vi "(Depricated) Dialog Sample.vi"(7 "Sample Line Control Ref":refnum<vi>, 8 "Error In":errorcluster, 11 "Caller-To-Actor Enqueuer":refnum<class "Message Enqueuer.lvclass">) -> (0 "Error Out":errorcluster, 1 "Sample Removed":bool, 3 "Cancelled?":bool)   [LabVIEW 2015]
doc: "Use this template to create a dialog box with event handling."
uses:
  <vilib>/ActorFramework/Message Enqueuer/Message Enqueuer.lvclass
  Controls/Ti Colors.ctl
panel:
  out "Color Box":u32(colorbox)
  in  "Remove Button":bool
  in  "Comment":string
  in  "Ti Cathode":i8 min=-1 max=39 step=1
  in  "Sample Name":string
  in  "Cancel":bool
  in  "OK":bool
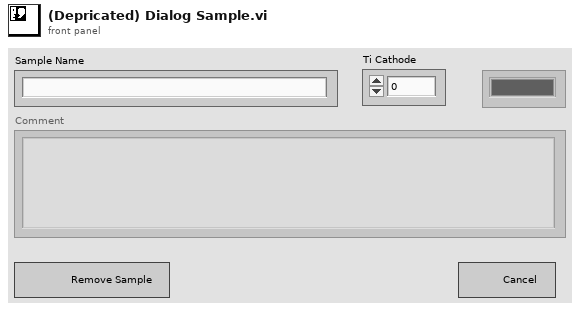
[diagram p1: front panel]
types:
  T1 = typedef "Ti Colors.ctl" = u32[]
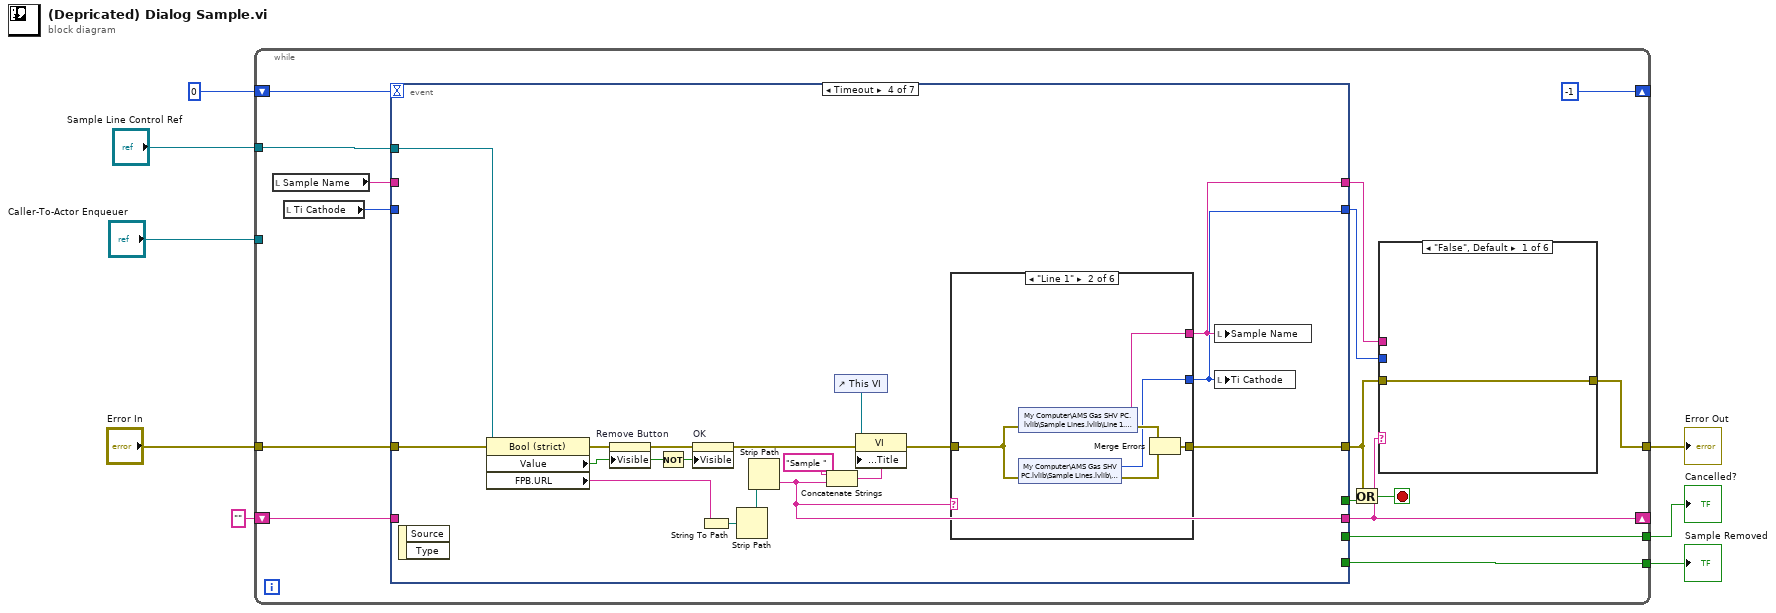
[diagram p0: block diagram]
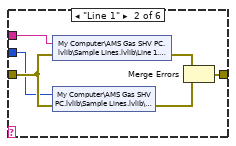
[diagram p2: hidden frame]
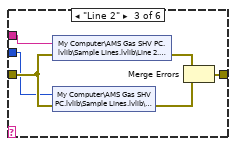
[diagram p3: hidden frame]
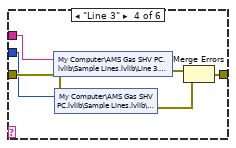
[diagram p4: hidden frame]
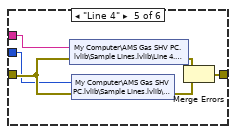
[diagram p5: hidden frame]
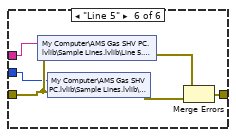
[diagram p6: hidden frame]
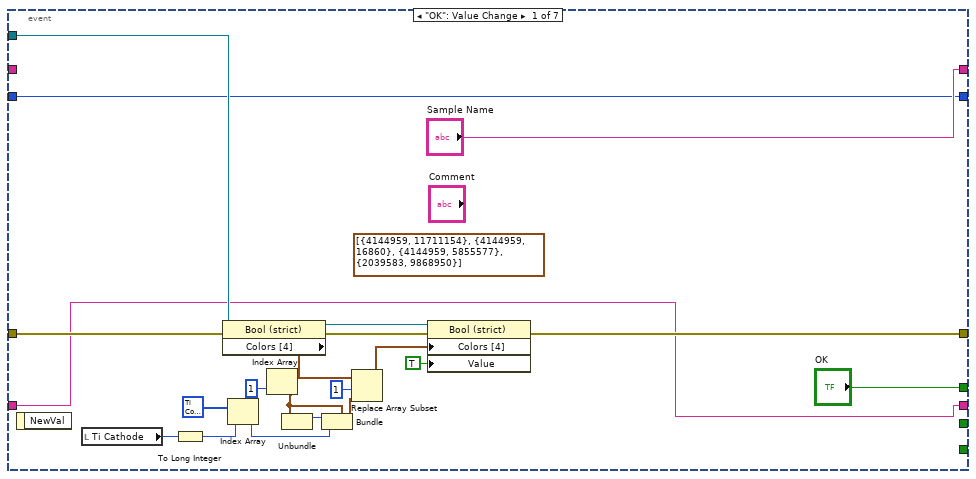
[diagram p7: hidden frame]
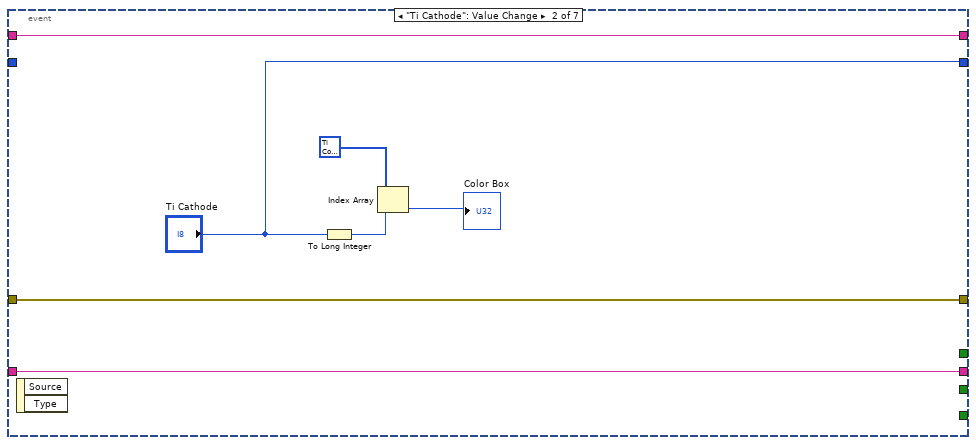
[diagram p8: hidden frame]
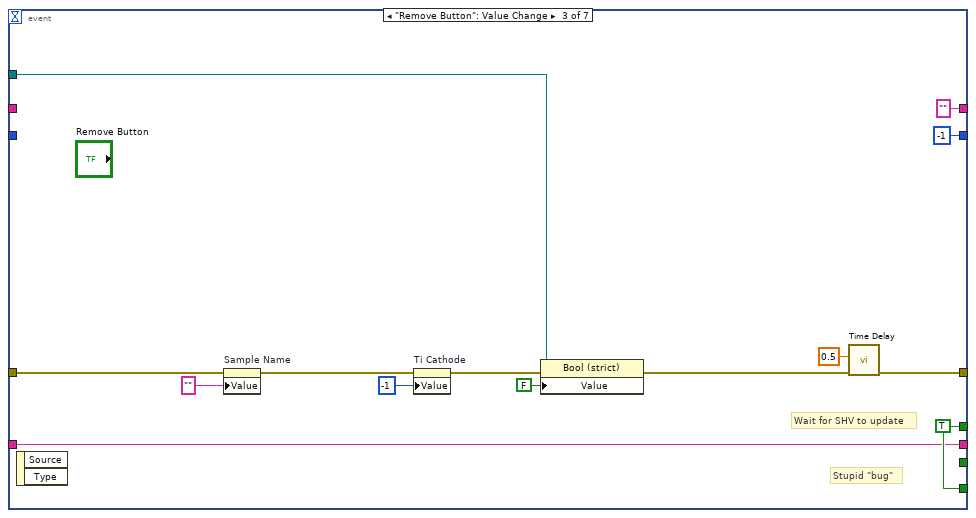
[diagram p9: hidden frame]
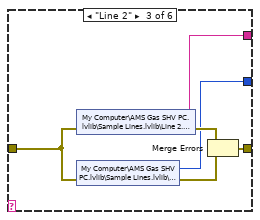
[diagram p11: hidden frame]
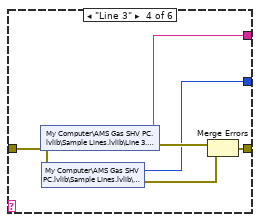
[diagram p12: hidden frame]
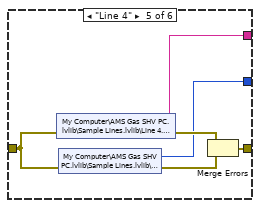
[diagram p13: hidden frame]
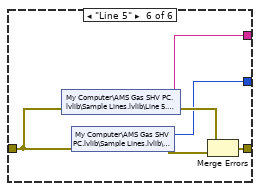
[diagram p14: hidden frame]
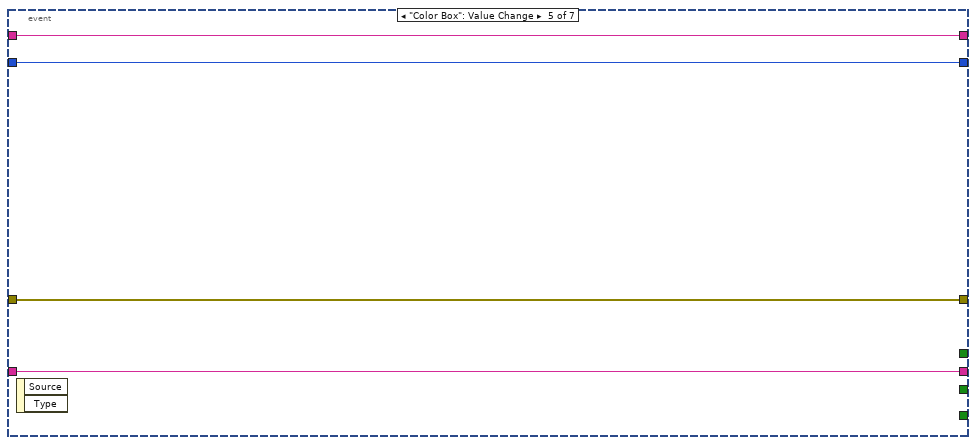
[diagram p15: hidden frame]
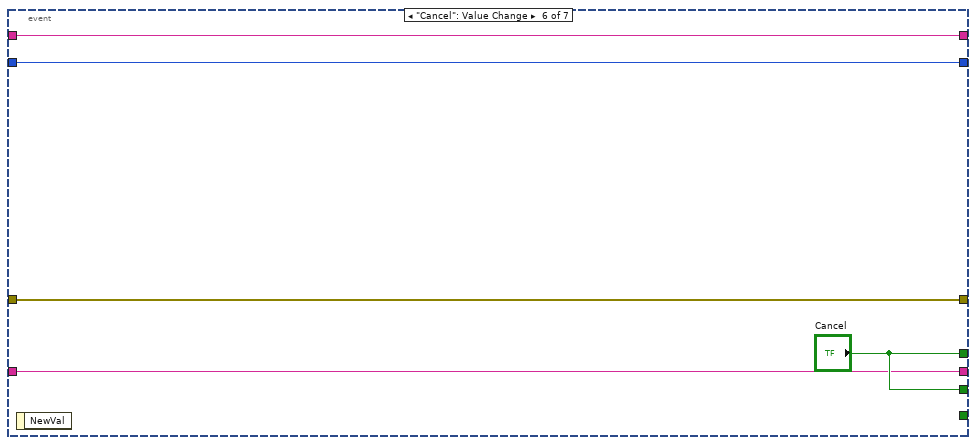
[diagram p16: hidden frame]
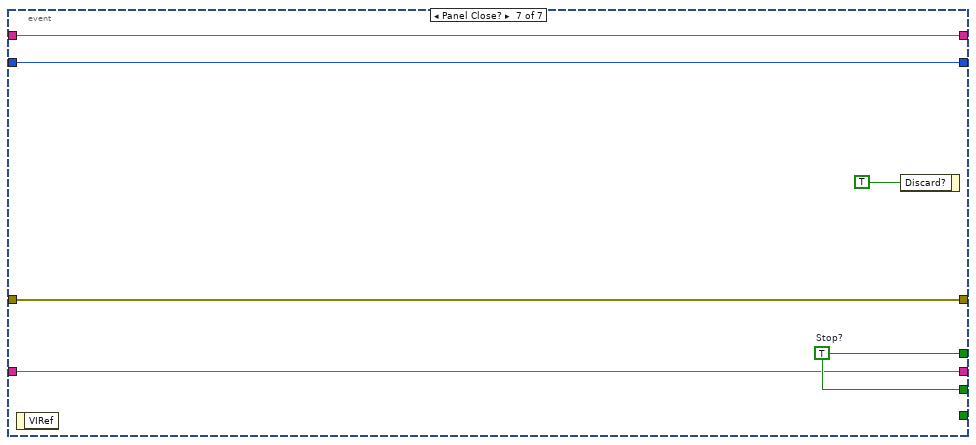
[diagram p17: hidden frame]
diagram:
  n1 = while {
    tunnel: "Error In" -> [w24]
    tunnel: "Caller-To-Actor Enqueuer" -> [_]
    tunnel: [w15] -> w7
    tunnel: "Sample Line Control Ref" -> [w23]
    shift-right: [-1] -> _
    shift-left: 0 -> [w20]
    tunnel: [w19] -> w4
    tunnel: [w17] -> w2
    shift-right: [w14] -> _
    shift-left: "" ("name") -> [w13]
    stop <- w21 stop-if-true
    n2 = local read "Sample Name"() -> (w12:string)
    n3 = local read "Ti Cathode"() -> (w11:i8)
    n4 = event shown="[3] Timeout" {
      selector: _ -> [_ _ _ _ _ _ _]
      dyn-events: _ -> [_ _ _ _ _ _ _]
      timeout: w20 -> [_ _ _ _ _ _ _]
      tunnel: ["OK" _ w89 _ _ "Cancel" w158] -> w22
      tunnel: w24 -> [w73 w80 w92 w112 w149 w154 w159]
      tunnel: [w75 w80 w94 w101 w149 w154 w159] -> w16
      tunnel: w23 -> [w71 _ w97 w113 _ _ _]
      tunnel: [_ _ _ _ _ "Cancel" w158] -> w19
      tunnel: [_ _ w89 _ _ _ _] -> w17
      tunnel: [w61 w79 w86 w100 w148 w152 w157] -> w14
      tunnel: w13 -> [w61 w79 w86 _ w148 w152 w157]
      tunnel: w12 -> [_ w78 _ _ w147 w151 w156]
      tunnel: w11 -> [w59 _ _ _ w146 w150 w155]
      tunnel: ["Sample Name" w78 "" ("Sample Name") w99 w147 w151 w156] -> w10
      tunnel: [w59 "Ti Cathode" i8 -1 ("Ti Cathode") w98 w146 w150 w155] -> w9
      event "OK": Value Change {
        (unwired) cluster{u32, u32}[] [{4144959, 11711154}, {4144959, 16860}, {4144959, 5855577}, {2039583, 9868950}] ("Colors [4]")
        n5 = event-data() -> ()  [unwired: 1 in, 1 out]
        n6 = local read "Ti Cathode"() -> (w65:i8)
        n7 = To Long Integer(number=w65) -> (32bit integer=w64:i32)
        n8 = property class="Bool (strict)"(reference=w71, error in=w73) -> (reference out=w70:refnum<vi>, error out=w72:errorcluster, "Colors [4]"=w62:cluster{u32, u32}[])
        n9 = Index Array(array=T1 [418898, 837796, 1256694, 1675592, 2094490, 2513388, 2932286, 3351184, 3770082, 4188980, 4607878, 5026776, 5445674, 5864572, 6283470, 6702368, 7121266, 7540164, 7959062, 8377960, 8796858, 9215756, 9634654, 10053552, 10472450, 10891348, 11310246, 11729144, 12148042, 12566940, 12985838, 13404736, 13823634, 14242532, 14661430, 15080328, 15499226, 15918124, 16337022, 16755920] ("output array 2"), index=w64) -> (element=w63:u32)
        n10 = Index Array(array=w62, index=1) -> (element=w67:cluster{u32, u32})
        n11 = Unbundle(w67) -> (w69:u32)  [unwired: 1 out]
        n12 = Bundle(cluster=w67, w69, w63) -> (w68:cluster{u32, u32})
        n13 = Replace Array Subset(array=w62, new element=w68, index=1) -> (w56:cluster{u32, u32}[])
        n14 = property class="Bool (strict)"(reference=w70, error in=w72, "Colors [4]"=w56, "Value"=TRUE) -> (error out=w75:errorcluster)  [unwired: 1 out]
      }
      event "Ti Cathode": Value Change {
        n15 = event-data() -> ()  [unwired: 1 in, 2 out]
        n16 = To Long Integer(number="Ti Cathode") -> (32bit integer=w82:i32)
        n17 = Index Array(array=T1 [418898, 837796, 1256694, 1675592, 2094490, 2513388, 2932286, 3351184, 3770082, 4188980, 4607878, 5026776, 5445674, 5864572, 6283470, 6702368, 7121266, 7540164, 7959062, 8377960, 8796858, 9215756, 9634654, 10053552, 10472450, 10891348, 11310246, 11729144, 12148042, 12566940, 12985838, 13404736, 13823634, 14242532, 14661430, 15080328, 15499226, 15918124, 16337022, 16755920] ("output array 2"), index=w82) -> (element=→"Color Box":u32)
      }
      event "Remove Button": Value Change {
        w89 = TRUE ("Stop?")
        # "Stupid \"bug\""
        # "Wait for SHV to update"
        n18 = event-data() -> ()  [unwired: 1 in, 2 out]
        n19 = property on="Sample Name" class="Str"(error in=w92, "Value"="" ("Sample Name")) -> (error out=w95:errorcluster)  [unwired: 1 in, 1 out]
        n20 = property on="Ti Cathode" class="DigNum (strict)"(error in=w95, "Value"=i8 -1 ("Value (Signaling)")) -> (error out=w91:errorcluster)  [unwired: 1 in, 1 out]
        n21 = property class="Bool (strict)"(reference=w97, error in=w91, "Value"=FALSE) -> (error out=w87:errorcluster)  [unwired: 1 out]
        n22 = call "Time Delay"("error in (no error)"=w87, "Delay Time (s)"=0.5) -> ("error out"=w94:errorcluster)  [unwired: 9 in]
      }
      event Timeout {
        n23 = event-data() -> ()  [unwired: 1 in, 2 out]
        n24 = property class="Bool (strict)"(reference=w113) -> ("Value"=w106:bool, "FPB.URL"=w110:string)  [unwired: 1 in, 2 out]
        n25 = property on="Remove Button" class="Bool"(error in=w112, "Visible"=w106) -> (error out=w107:errorcluster)  [unwired: 1 in, 1 out]
        n26 = Not(x=w106) -> (.not. x?=w105:bool)
        n27 = property on="OK" class="Bool"(error in=w107, "Visible"=w105) -> (error out=w104:errorcluster)  [unwired: 1 in, 1 out]
        n28 = String To Path(string=w110) -> (path=w114:path)
        n29 = Strip Path(path=w114) -> (stripped path=w103:path)  [unwired: 1 out]
        n30 = Strip Path(path=w103) -> (name=w100:string)  [unwired: 1 out]
        n31 = Concatenate Strings("Sample " ("string"), w100) -> (w109:string)
        n32 = control-ref of="This VI"() -> (w111:refnum<vi>)
        n33 = property class="VI"(reference=w111, error in=w104, "Front Panel.Title"=w109) -> (error out=w102:errorcluster)  [unwired: 1 out]
        n34 = case shown="\"Line 1\"" w100 {
          tunnel: w102 -> [w115 w121 w127 w132 w138 w144]
          tunnel: [w115 w120 w126 w133 w139 w145] -> w101
          tunnel: [_ w117 w123 w129 w135 w141] -> w99
          tunnel: [_ w116 w122 w128 w134 w140] -> w98
          frame "False", Default {
          }
          frame "Line 1" {
            n35 = shared-variable "My Computer\\AMS Gas SHV PC.lvlib\\Sample Lines.lvlib\\Line 1.lvlib\\Sample Name"(error in=w121) -> (w117:string, error out=w118:errorcluster)
            n36 = shared-variable "My Computer\\AMS Gas SHV PC.lvlib\\Sample Lines.lvlib\\Line 1.lvlib\\Ti Cathode"(error in=w121) -> (w116:i8, error out=w119:errorcluster)
            n37 = Merge Errors(w118, w119) -> (w120:errorcluster)
          }
          frame "Line 2" {
            n38 = shared-variable "My Computer\\AMS Gas SHV PC.lvlib\\Sample Lines.lvlib\\Line 2.lvlib\\Sample Name"(error in=w127) -> (w123:string, error out=w124:errorcluster)
            n39 = shared-variable "My Computer\\AMS Gas SHV PC.lvlib\\Sample Lines.lvlib\\Line 2.lvlib\\Ti Cathode"(error in=w127) -> (w122:i8, error out=w125:errorcluster)
            n40 = Merge Errors(w124, w125) -> (w126:errorcluster)
          }
          frame "Line 3" {
            n41 = shared-variable "My Computer\\AMS Gas SHV PC.lvlib\\Sample Lines.lvlib\\Line 3.lvlib\\Sample Name"(error in=w132) -> (w129:string, error out=w130:errorcluster)
            n42 = shared-variable "My Computer\\AMS Gas SHV PC.lvlib\\Sample Lines.lvlib\\Line 3.lvlib\\Ti Cathode"(error in=w132) -> (w128:i8, error out=w131:errorcluster)
            n43 = Merge Errors(w130, w131) -> (w133:errorcluster)
          }
          frame "Line 4" {
            n44 = shared-variable "My Computer\\AMS Gas SHV PC.lvlib\\Sample Lines.lvlib\\Line 4.lvlib\\Sample Name"(error in=w138) -> (w135:string, error out=w137:errorcluster)
            n45 = shared-variable "My Computer\\AMS Gas SHV PC.lvlib\\Sample Lines.lvlib\\Line 4.lvlib\\Ti Cathode"(error in=w138) -> (w134:i8, error out=w136:errorcluster)
            n46 = Merge Errors(w137, w136) -> (w139:errorcluster)
          }
          frame "Line 5" {
            n47 = shared-variable "My Computer\\AMS Gas SHV PC.lvlib\\Sample Lines.lvlib\\Line 5.lvlib\\Sample Name"(error in=w144) -> (w141:string, error out=w142:errorcluster)
            n48 = shared-variable "My Computer\\AMS Gas SHV PC.lvlib\\Sample Lines.lvlib\\Line 5.lvlib\\Ti Cathode"(error in=w144) -> (w140:i8, error out=w143:errorcluster)
            n49 = Merge Errors(w142, w143) -> (w145:errorcluster)
          }
        }
        n50 = local write "Sample Name"(w99) -> ()
        n51 = local write "Ti Cathode"(w98) -> ()
      }
      event "Color Box": Value Change {
        n52 = event-data() -> ()  [unwired: 1 in, 2 out]
      }
      event "Cancel": Value Change {
        n53 = event-data() -> ()  [unwired: 1 in, 1 out]
      }
      event Panel Close? {
        w158 = TRUE  # Stop?
        n54 = event-data() -> ()  [unwired: 1 in, 1 out]
        n55 = event-data("Discard?"=TRUE) -> ()  [unwired: 1 in, 1 out]
      }
    }
    n56 = Or(x=w16, y=w22) -> (x .or. y?=w21:bool)
    n57 = case shown="\"False\", Default" w14 {
      tunnel: w16 -> [w25 w31 w37 w42 w46 w52]
      tunnel: [w25 w30 w36 w43 w49 w55] -> w15
      tunnel: w10 -> [_ w27 w33 w39 w45 w50]
      tunnel: w9 -> [_ w26 w32 w38 w44 w51]
      frame "False", Default {
      }
      frame "Line 1" {
        n58 = shared-variable "My Computer\\AMS Gas SHV PC.lvlib\\Sample Lines.lvlib\\Line 1.lvlib\\Sample Name"(w27, error in=w31) -> (error out=w28:errorcluster)
        n59 = shared-variable "My Computer\\AMS Gas SHV PC.lvlib\\Sample Lines.lvlib\\Line 1.lvlib\\Ti Cathode"(w26, error in=w31) -> (error out=w29:errorcluster)
        n60 = Merge Errors(w28, w29) -> (w30:errorcluster)
      }
      frame "Line 2" {
        n61 = shared-variable "My Computer\\AMS Gas SHV PC.lvlib\\Sample Lines.lvlib\\Line 2.lvlib\\Sample Name"(w33, error in=w37) -> (error out=w34:errorcluster)
        n62 = shared-variable "My Computer\\AMS Gas SHV PC.lvlib\\Sample Lines.lvlib\\Line 2.lvlib\\Ti Cathode"(w32, error in=w37) -> (error out=w35:errorcluster)
        n63 = Merge Errors(w34, w35) -> (w36:errorcluster)
      }
      frame "Line 3" {
        n64 = shared-variable "My Computer\\AMS Gas SHV PC.lvlib\\Sample Lines.lvlib\\Line 3.lvlib\\Sample Name"(w39, error in=w42) -> (error out=w40:errorcluster)
        n65 = shared-variable "My Computer\\AMS Gas SHV PC.lvlib\\Sample Lines.lvlib\\Line 3.lvlib\\Ti Cathode"(w38, error in=w42) -> (error out=w41:errorcluster)
        n66 = Merge Errors(w40, w41) -> (w43:errorcluster)
      }
      frame "Line 4" {
        n67 = shared-variable "My Computer\\AMS Gas SHV PC.lvlib\\Sample Lines.lvlib\\Line 4.lvlib\\Sample Name"(w45, error in=w46) -> (error out=w48:errorcluster)
        n68 = shared-variable "My Computer\\AMS Gas SHV PC.lvlib\\Sample Lines.lvlib\\Line 4.lvlib\\Ti Cathode"(w44, error in=w46) -> (error out=w47:errorcluster)
        n69 = Merge Errors(w48, w47) -> (w49:errorcluster)
      }
      frame "Line 5" {
        n70 = shared-variable "My Computer\\AMS Gas SHV PC.lvlib\\Sample Lines.lvlib\\Line 5.lvlib\\Sample Name"(w50, error in=w52) -> (error out=w53:errorcluster)
        n71 = shared-variable "My Computer\\AMS Gas SHV PC.lvlib\\Sample Lines.lvlib\\Line 5.lvlib\\Ti Cathode"(w51, error in=w52) -> (error out=w54:errorcluster)
        n72 = Merge Errors(w53, w54) -> (w55:errorcluster)
      }
    }
  }
  "Error Out" <- w7
  "Cancelled?" <- w4
  "Sample Removed" <- w2
